vi "Dialog_Macro Launch Options.vi"(8 "error in (no error)":errorcluster) -> (0 "error out":errorcluster, 3 "Load Temp?":bool)   [LabVIEW 2012]
doc: "SciScan 1.2 160622"
panel:
  in  "OK Button":bool
  in  "Please select your launch option":T1(radio)
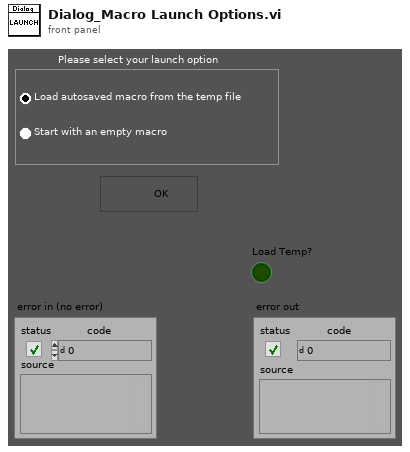
[diagram p1: front panel]
types:
  T1 = enum32{"Load autosaved macro from the temp file", "Start with an empty macro"}
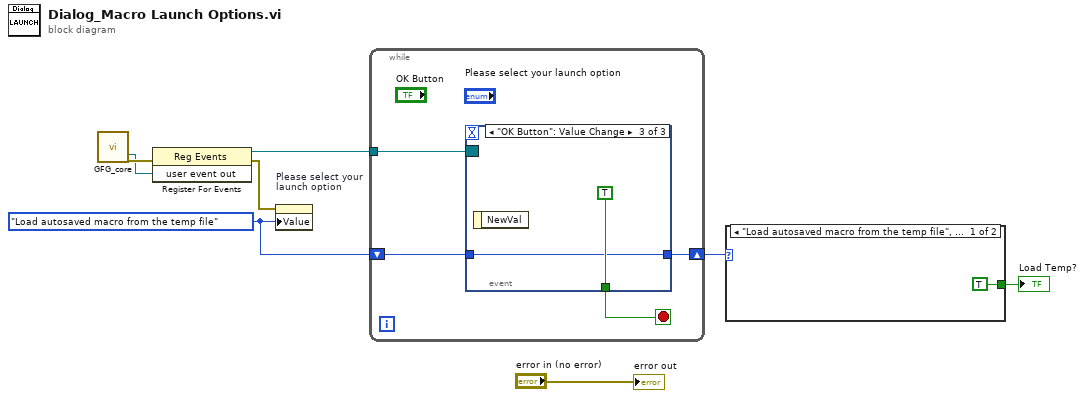
[diagram p0: block diagram]
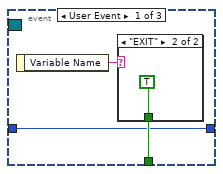
[diagram p3: hidden frame]
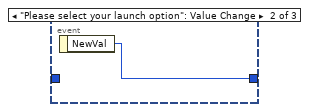
[diagram p5: hidden frame]
diagram:
  w3 = T1."Load autosaved macro from the temp file" ("Radio Buttons")
  n1 = call "GFG_core.vi"() -> ("user event out"=w7:refnum<user-event>, "error out"=w8:errorcluster)  [unwired: 13 in, 5 out]
  n2 = register-events(error in=w8, w7) -> (reference out=w6:refnum<event-registration>, error out=w5:errorcluster)  [unwired: 1 in]
  n3 = property on="Please select your launch option" class="RadioBtnsControl (strict)"(error in=w5, "Value"=w3) -> ()  [unwired: 1 in, 2 out]
  n4 = while {
    tunnel: w6 -> [w12]
    shift-right: [w10] -> w2
    shift-left: w3 -> [w9]
    stop <- w11 stop-if-true
    n5 = event shown="[2] \"OK Button\": Value Change" {
      selector: w12 -> [_ _ _]
      dyn-events: _ -> [_ _ _]
      timeout: _ -> [_ _ _]
      tunnel: [w14 _ TRUE] -> w11
      tunnel: [w13 w17 w18] -> w10
      tunnel: w9 -> [w13 _ w18]
      event User Event {
        n6 = event-data() -> ("Variable Name"=w15:string)  [unwired: 1 in]
        n7 = case shown="\"EXIT\"" w15 {
          tunnel: [_ TRUE] -> w14
          frame "False", Default {
          }
          frame "EXIT" {
          }
        }
      }
      event "Please select your launch option": Value Change {
        n8 = event-data() -> ("NewVal"=w17:T1)  [unwired: 1 in]
      }
      event "OK Button": Value Change {
        n9 = event-data() -> ()  [unwired: 1 in, 1 out]
      }
    }
  }
  n10 = case shown="\"Load autosaved macro from the temp file\", Default" w2 {
    tunnel: [TRUE _] -> w1
    frame "Load autosaved macro from the temp file", Default {
    }
    frame "Start with an empty macro" {
    }
  }
  "Load Temp?" <- w1
  "error out" <- "error in (no error)"
